vi "SENS_SEGM_ARB_ON_OFF.vi"(0 "VISA IN":refnum<visa-resource-name>, 1 "ARB ON/OFF":bool, 5 "error in":errorcluster, 7 "Channel":i32) -> (14 "VISA Out":refnum<visa-resource-name>, 19 "error out":errorcluster)   [LabVIEW 2018, in "PNA-X.lvlib"]
doc: "SENSe<cnum>:SEGMent:ARBitrary <ON | OFF> \n1805\n\n(Read-Write) Enables you to setup a segment sweep with arbitrary frequencies. The start and stop \nfrequencies of each segment can overlap other segments. Also, each segment can have a start \nfrequency that is greater than its stop frequency which causes a reverse sweep over that segment. \nLearn more about Arbitrary Segment Sweep. \nParameters \n<cnum> Any existing channel number. If unspecified, value is set to 1. \n<ON | OFF> ON (or 1) - Allows the setup of arbitrary segment sweep. \nOFF (or 0) - Prevents the setup of arbitrary segment sweep. \nExamples SENS:SEGM:ARB ON \nsense2:segment:arbitrary off \nQuery Syntax SENSe<cnum>:SEGMent:ARBitrary? \nReturn Type Boolean (1 = ON, 0 = OFF) \nDefault OFF"
uses:
  PNA-X.lvlib
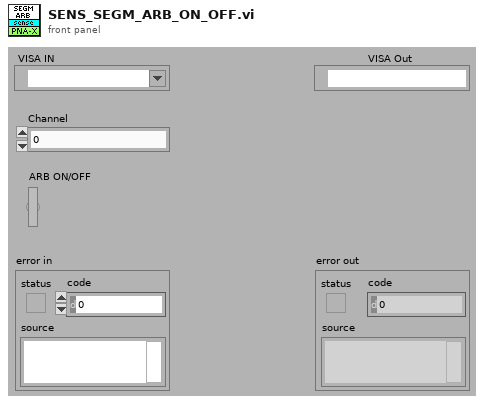
[diagram p1: front panel]
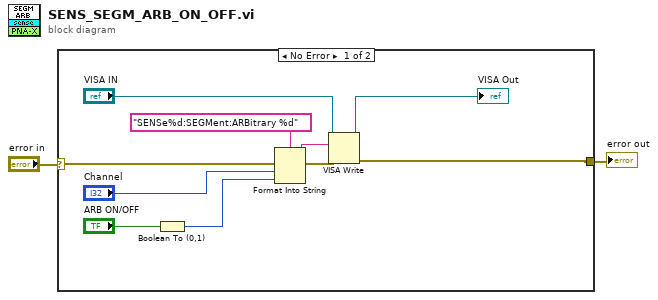
[diagram p0: block diagram]
diagram:
  n1 = case shown="No Error" "error in" {
    selector: "error in" -> [w12 w13]
    tunnel: [w7 w13] -> w1
    frame No Error {
      n2 = Boolean To (0,1)(Boolean="ARB ON/OFF") -> (0, 1=w3:i16)
      n3 = Format Into String(format string="SENSe%d:SEGMent:ARBitrary %d" ("Cmdline"), error in=w12, "Channel", w3) -> (resulting string=w10:string, error out=w11:errorcluster)  [unwired: 1 in]
      n4 = VISA Write(VISA resource name="VISA IN", write buffer=w10, error in (no error)=w11) -> (VISA resource name out=→"VISA Out":refnum<visa-resource-name>, error out=w7:errorcluster)  [unwired: 1 out]
    }
    frame Error {
    }
  }
  "error out" <- w1
